vi "13_1.vi"() -> ()   [LabVIEW 2018]
panel:
  out "x*y":dbl
  in  "Input":string
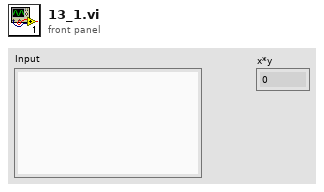
[diagram p1: front panel]
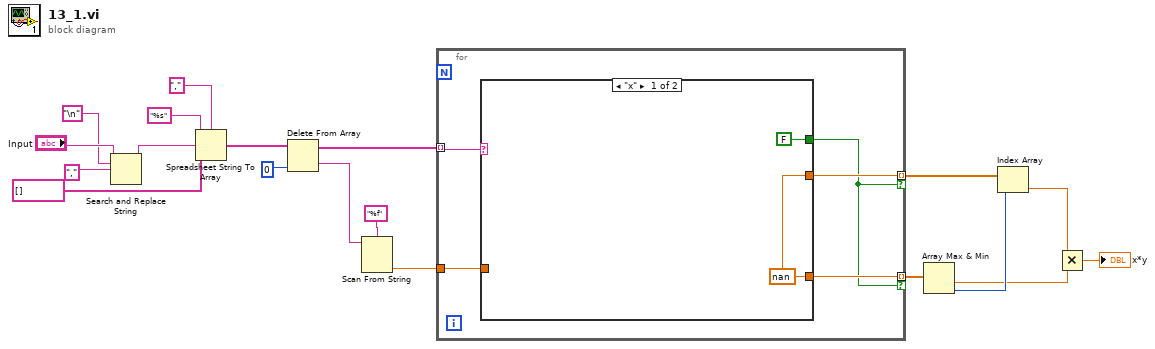
[diagram p0: block diagram]
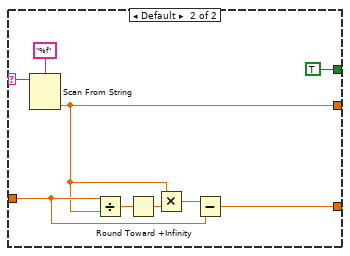
[diagram p2: hidden frame]
diagram:
  n1 = Search and Replace String(input string="Input", search string="\n", replace string=",") -> (result string=w14:string)  [unwired: 5 in, 3 out]
  n2 = Spreadsheet String To Array(delimiter (Tab)=",", format string="%s", spreadsheet string=w14, array type (2D Dbl)=string[] []) -> (array=w11:string[])
  n3 = Delete From Array(array=w11, index=0) -> (deleted portion=w9:string, array with subset deleted=w8:string[])  [unwired: 1 in]
  n4 = Scan From String(format string="%f", input string=w9) -> (output 1=w7:dbl)  [unwired: 3 in, 3 out]
  n5 = for {
    tunnel: w8 -> [w24] mode=indexing
    tunnel: w7 -> [w23]
    tunnel: [w22] -> w5 mode=indexing if=w20
    tunnel: [w21] -> w6 mode=indexing if=w20
    n6 = case shown="\"x\"" w24 {
      selector: w24 -> [_ w34]
      tunnel: w23 -> [_ w30]
      tunnel: [w25 w29] -> w21
      tunnel: [w25 w28] -> w22
      tunnel: [FALSE TRUE] -> w20
      frame "x" {
        w25 = nan
      }
      frame Default {
        n7 = Scan From String(format string="%f", input string=w34) -> (output 1=w28:dbl)  [unwired: 3 in, 3 out]
        n8 = Divide(x=w30, y=w28) -> (x/y=w33:dbl)
        n9 = Round Toward +Infinity(x=w33) -> (ceil(x): smallest int >= x=w32:dbl)
        n10 = Multiply(x=w28, y=w32) -> (x*y=w31:dbl)
        n11 = Subtract(x=w31, y=w30) -> (x-y=w29:dbl)
      }
    }
  }
  n12 = Array Max & Min(array=w6) -> (min value=w3:dbl, min index (indices)=w4:i32)  [unwired: 2 out]
  n13 = Index Array(array=w5, index=w4) -> (element=w2:dbl)
  n14 = Multiply(x=w2, y=w3) -> (x*y=→"x*y":dbl)
